vi "Create.vi"(8 "error in (no error)":errorcluster, 10 "Name":string, 11 "object in":refnum<class "EventMsg.lvclass">) -> (0 "error out":errorcluster, 2 "EMSG_EvRef":refnum<user-event>, 3 "object out":refnum<class "EventMsg.lvclass">)   [LabVIEW 2014, in "EventMsg.lvclass"]
doc: "Create a event reference and store name to refer to this event reference.\n\nThis is useful by using fire to all or fire (this refer by name)"
uses:
  EventMsg.lvclass
  EventMsg.lvclass/EventMsg.ctl
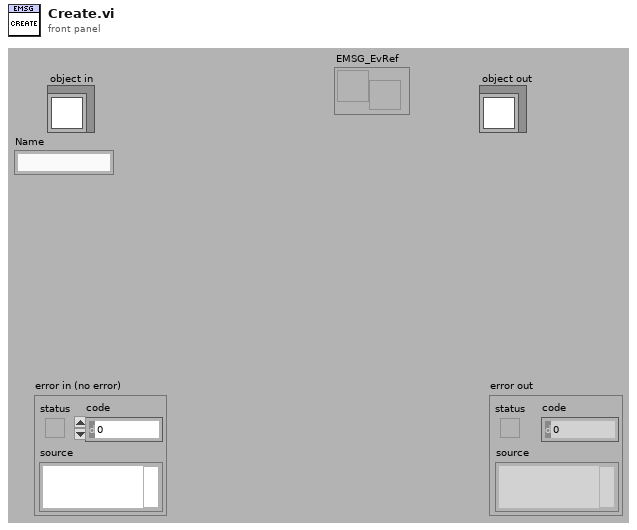
[diagram p1: front panel]
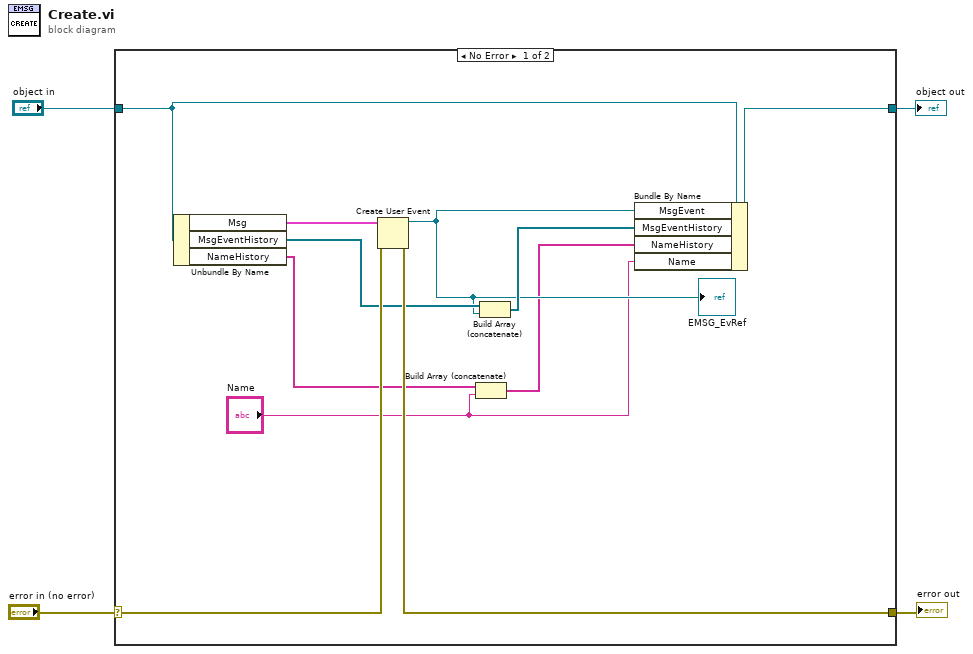
[diagram p0: block diagram]
diagram:
  n1 = case shown="No Error" "error in (no error)" {
    selector: "error in (no error)" -> [w15 w17]
    tunnel: [w14 w17] -> w3
    tunnel: [w12 w16] -> w1
    tunnel: "object in" -> [w11 w16]
    frame No Error {
      n2 = Unbundle By Name(w11) -> ("Msg"=w13:cluster{"Msg":string, "Data":variant}, "MsgEventHistory"=w10:refnum<user-event>[], "NameHistory"=w7:string[])
      n3 = Create User Event(user event datatype=w13, error in=w15) -> (user event=w8:refnum<user-event>, error out=w14:errorcluster)
      "EMSG_EvRef" <- w8
      n4 = Build Array (concatenate)(w7, "Name") -> (w6:string[])
      n5 = Build Array (concatenate)(w10, w8) -> (w9:refnum<user-event>[])
      n6 = Bundle By Name(cluster=w11, "MsgEvent"=w8, "MsgEventHistory"=w9, "NameHistory"=w6, "Name"="Name") -> (w12:refnum<class "EventMsg.lvclass">)
    }
    frame Error {
    }
  }
  "error out" <- w3
  "object out" <- w1
